vi "Unpack For Grpc.vi"(7 "Results? (Config)":bool, 8 "error in (no error)":errorcluster, 10 "Any":T1, 11 "gRPCid":T2) -> (0 "error out":errorcluster, 2 "Data Value":variant)   [LabVIEW 2020, in "MeasurementLink Measurement Template.lvlib"]
uses:
  MeasurementLink Measurement Template.lvlib
  <vilib>/gRPC/LabVIEW gRPC Library/Shared/grpcId.ctl
  <vilib>/gRPC/LabVIEW gRPC Library/Shared/Any.ctl
  Measurement Results.ctl
  Measurement Configuration.ctl
  <vilib>/gRPC/LabVIEW gRPC Library/Server API/Translate Protobuf Error.vi
  <vilib>/AdvancedString/1D String Array to Delimited String.vi
  <vilib>/gRPC/LabVIEW gRPC Library/Server API/Server/Get Server DLL Path.vi
  2ea427b1-48cb-44ca-aad2-ce8ea2327057.vi
  53afc063-6da3-45f4-9d70-8055d1ba642d.vi
  <vilib>/gRPC/LabVIEW gRPC Library/grpc-lvsupport-release.lvlib
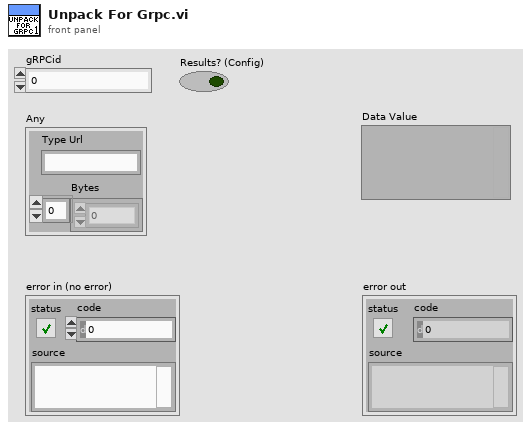
[diagram p1: front panel]
types:
  T1 = typedef "grpc-lvsupport-release.lvlib/Any.ctl" = cluster{"Type Url":string, "Bytes":u8[]}
  T2 = typedef "grpc-lvsupport-release.lvlib/grpcId.ctl" = u64
  T3 = typedef "MeasurementLink Measurement Template.lvlib/Measurement Results.ctl" = cluster{"Array out":dbl[]}
  T4 = typedef "MeasurementLink Measurement Template.lvlib/Measurement Configuration.ctl" = cluster{"Array in":dbl[]}
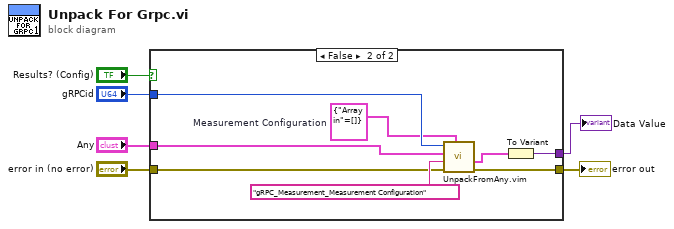
[diagram p0: block diagram]
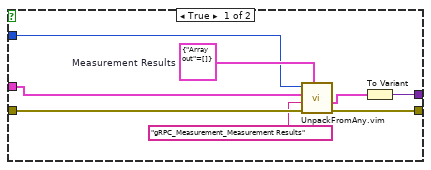
[diagram p2: hidden frame]
diagram:
  n1 = case shown="False" "Results? (Config)" {
    tunnel: "error in (no error)" -> [w12 w19]
    tunnel: "Any" -> [w10 w17]
    tunnel: "gRPCid" -> [w9 w20]
    tunnel: [w14 w22] -> w4
    tunnel: [w7 w15] -> w1
    frame True {
      w13 = T3 {"Array out"=[]}  # Measurement Results
      n2 = call "UnpackFromAny.vim"("Data Type"=w13, "error in"=w12, "Message Type"="gRPC_Measurement_Measurement Results", "Any"=w10, "gRPCid in"=w9) -> ("error out"=w14:errorcluster, "Unpacked Value"=w8:T3)  [unwired: 4 in, 1 out]
      n3 = To Variant(anything=w8) -> (Variant=w7:variant)
    }
    frame False {
      w18 = T4 {"Array in"=[]}  # Measurement Configuration
      n4 = call "UnpackFromAny.vim"("Data Type"=w18, "error in"=w19, "Message Type"="gRPC_Measurement_Measurement Configuration", "Any"=w17, "gRPCid in"=w20) -> ("error out"=w22:errorcluster, "Unpacked Value"=w16:T4)  [unwired: 4 in, 1 out]
      n5 = To Variant(anything=w16) -> (Variant=w15:variant)
    }
  }
  "error out" <- w4
  "Data Value" <- w1
